vi "Guitar SubviUpdated.vi"(0 "error out":errorcluster, 1 "Image Dst Out":T2) -> (11 "Orange Guitar LED":bool, 13 "Red Guitar LED":bool, 15 "Green Guitar LED":bool, 23 "Blue Guitar LED":bool, 24 "Yellow Guitar LED":bool)   [LabVIEW 2009]
uses:
  <vilib>/vision/Image Controls.llb/IMAQ Image.ctl
  <vilib>/Analysis/3filter.llb/Filter Passband Type.ctl
  <vilib>/Analysis/3filter.llb/Butterworth Filter (DBL).vi
  <vilib>/Analysis/NI_AALBase.lvlib
  <vilib>/vision/NI_Vision_Development_Module.lvlib
panel:
  in  "Yellow Guitar":T1={"Global Rectangle"=[40, 272, 657, 396], "Contours"=[{"ID"=enum."External", "Type"=3, "Coordinates"=[40, 272, 657, 396]}]} {"Contours"."Type" items=["No Selection", "Point", "Line", "Rectangle", "Oval", "Polygon", "Freehand Region", "Annulus", "Unused2", "Unused3", "Broken Line", "Freehand Line", "Rotated Rectangle"]}
  in  "Red Guitar":T1={"Global Rectangle"=[40, 272, 657, 396], "Contours"=[{"ID"=enum."External", "Type"=3, "Coordinates"=[40, 272, 657, 396]}]} {"Contours"."Type" items=["No Selection", "Point", "Line", "Rectangle", "Oval", "Polygon", "Freehand Region", "Annulus", "Unused2", "Unused3", "Broken Line", "Freehand Line", "Rotated Rectangle"]}
  in  "Orange Guitar":T1={"Global Rectangle"=[40, 272, 657, 396], "Contours"=[{"ID"=enum."External", "Type"=3, "Coordinates"=[40, 272, 657, 396]}]} {"Contours"."Type" items=["No Selection", "Point", "Line", "Rectangle", "Oval", "Polygon", "Freehand Region", "Annulus", "Unused2", "Unused3", "Broken Line", "Freehand Line", "Rotated Rectangle"]}
  in  "Green Guitar":T1={"Global Rectangle"=[40, 272, 657, 396], "Contours"=[{"ID"=enum."External", "Type"=3, "Coordinates"=[40, 272, 657, 396]}]} {"Contours"."Type" items=["No Selection", "Point", "Line", "Rectangle", "Oval", "Polygon", "Freehand Region", "Annulus", "Unused2", "Unused3", "Broken Line", "Freehand Line", "Rotated Rectangle"]}
  in  "Blue Guitar":T1={"Global Rectangle"=[40, 272, 657, 396], "Contours"=[{"ID"=enum."External", "Type"=3, "Coordinates"=[40, 272, 657, 396]}]} {"Contours"."Type" items=["No Selection", "Point", "Line", "Rectangle", "Oval", "Polygon", "Freehand Region", "Annulus", "Unused2", "Unused3", "Broken Line", "Freehand Line", "Rotated Rectangle"]}
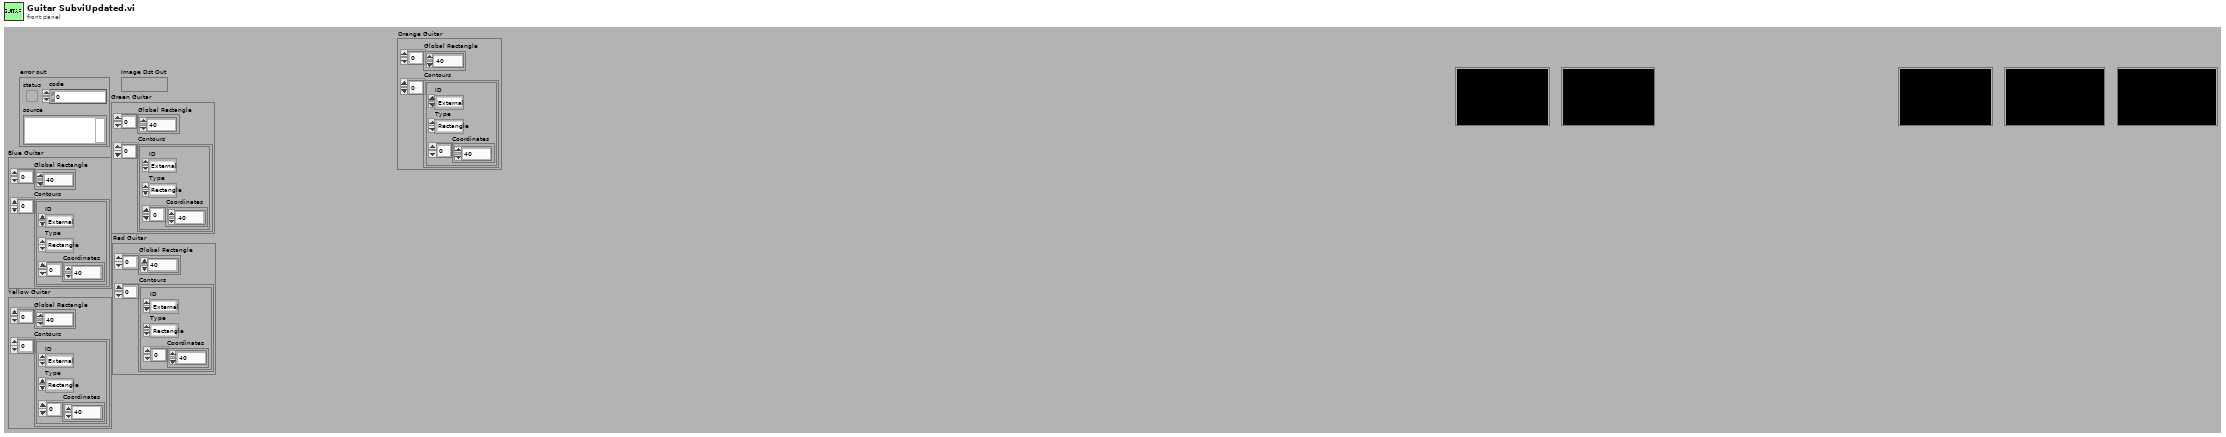
[diagram p1: front panel]
types:
  T1 = cluster{"Global Rectangle":i32[], "Contours":cluster{"ID":enum32{"External", "Internal"}, "Type":u32, "Coordinates":i32[]}[]}
  T2 = typedef "IMAQ Image.ctl" = refnum<image>
  T3 = typedef "NI_AALBase.lvlib/Filter Passband Type.ctl" = enum32{"Lowpass", "Highpass", "Bandpass", "Bandstop"}
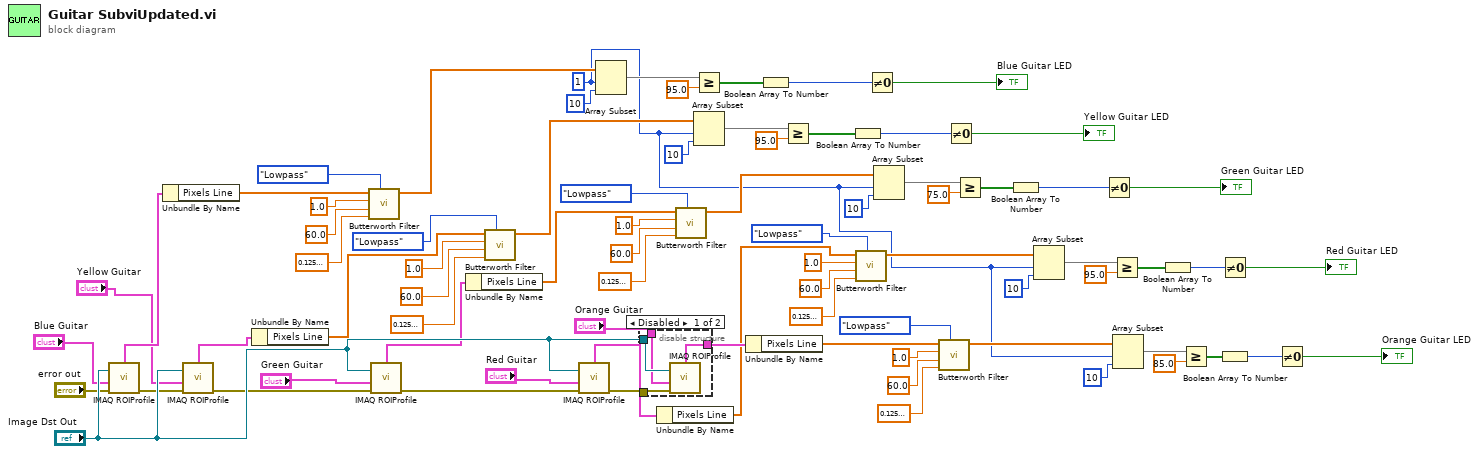
[diagram p0: block diagram]
diagram:
  w6 = 1 ("index")
  n1 = call "IMAQ ROIProfile"("error in (no error)"="error out", "ROI Descriptor"="Blue Guitar", "Image"="Image Dst Out") -> ("error out"=w47:errorcluster, "ROI Graph"=w46:cluster{"x0":sgl, "dx":sgl, "Pixels Line":sgl[]})  [unwired: 4 out]
  n2 = Unbundle By Name(w46) -> ("Pixels Line"=w67:sgl[])
  n3 = call "IMAQ ROIProfile"("error in (no error)"=w47, "ROI Descriptor"="Yellow Guitar", "Image"="Image Dst Out") -> ("error out"=w19:errorcluster, "ROI Graph"=w50:cluster{"x0":sgl, "dx":sgl, "Pixels Line":sgl[]})  [unwired: 4 out]
  n4 = Unbundle By Name(w50) -> ("Pixels Line"=w53:sgl[])
  n5 = call-poly <vilib>:"Butterworth Filter.vi"("filter type"=Filter_Passband_Type."Lowpass", "low cutoff freq: fl"=0.12500000000000006 ("low 3"), "high cutoff freq: fh"=60.0 ("high 14"), "sampling freq: fs"=1.0 ("sampling  9"), "X"=w67) -> ("Filtered X"=w33:dbl[])  [unwired: 3 in, 1 out]
  n6 = call "IMAQ ROIProfile"("error in (no error)"=w19, "ROI Descriptor"="Green Guitar", "Image"="Image Dst Out") -> ("error out"=w20:errorcluster, "ROI Graph"=w44:cluster{"x0":sgl, "dx":sgl, "Pixels Line":sgl[]})  [unwired: 4 out]
  n7 = Unbundle By Name(w44) -> ("Pixels Line"=w41:sgl[])
  n8 = call-poly <vilib>:"Butterworth Filter.vi"("filter type"=Filter_Passband_Type."Lowpass", "low cutoff freq: fl"=0.12500000000000006 ("low  12"), "high cutoff freq: fh"=60.0 ("high 13"), "sampling freq: fs"=1.0 ("sampling 12"), "X"=w53) -> ("Filtered X"=w49:dbl[])  [unwired: 3 in, 1 out]
  n9 = call "IMAQ ROIProfile"("error in (no error)"=w20, "ROI Descriptor"="Red Guitar", "Image"="Image Dst Out") -> ("error out"=w71:errorcluster, "ROI Graph"=w22:cluster{"x0":sgl, "dx":sgl, "Pixels Line":sgl[]})  [unwired: 4 out]
  n10 = Array Subset(array=w33, index=w6, length=10) -> (w62:dbl[])
  n11 = disable-structure shown="Disabled" {
    disable-tunnel: [w81 _] -> w72
    disable-tunnel: w71 -> [w80 _]
    disable-tunnel: "Image Dst Out" -> [w79 _]
    disable-tunnel: "Orange Guitar" -> [w78 _]
    frame #0 {
      n12 = call "IMAQ ROIProfile"("error in (no error)"=w80, "ROI Descriptor"=w78, "Image"=w79) -> ("ROI Graph"=w81:cluster{"x0":sgl, "dx":sgl, "Pixels Line":sgl[]})  [unwired: 5 out]
    }
    frame #1 {
    }
  }
  n13 = Unbundle By Name(w22) -> ("Pixels Line"=w25:sgl[])
  n14 = call-poly <vilib>:"Butterworth Filter.vi"("filter type"=Filter_Passband_Type."Lowpass", "low cutoff freq: fl"=0.12500000000000006 ("low  11"), "high cutoff freq: fh"=60.0 ("high 12"), "sampling freq: fs"=1.0 ("sampling 11"), "X"=w41) -> ("Filtered X"=w45:dbl[])  [unwired: 3 in, 1 out]
  n15 = Greater Or Equal?(x=w62, y=95.0) -> (x >= y?=w7:bool[])
  n16 = Array Subset(array=w49, index=w6, length=10) -> (w58:dbl[])
  n17 = Unbundle By Name(w72) -> ("Pixels Line"=w15:sgl[])
  n18 = Boolean Array To Number(Boolean array=w7) -> (number=w60:u32)
  n19 = Greater Or Equal?(x=w58, y=95.0) -> (x >= y?=w56:bool[])
  n20 = Boolean Array To Number(Boolean array=w56) -> (number=w55:u32)
  n21 = call-poly <vilib>:"Butterworth Filter.vi"("filter type"=Filter_Passband_Type."Lowpass", "low cutoff freq: fl"=0.12500000000000006 ("low  10"), "high cutoff freq: fh"=60.0 ("high 11"), "sampling freq: fs"=1.0 ("sampling 10"), "X"=w25) -> ("Filtered X"=w21:dbl[])  [unwired: 3 in, 1 out]
  n22 = Not Equal To 0?(x=w60) -> (x != 0?=→"Blue Guitar LED":bool)
  n23 = Array Subset(array=w45, index=w6, length=10) -> (w36:dbl[])
  n24 = call-poly <vilib>:"Butterworth Filter.vi"("filter type"=Filter_Passband_Type."Lowpass", "low cutoff freq: fl"=0.12500000000000006 ("low  9"), "high cutoff freq: fh"=60.0 ("high 10"), "sampling freq: fs"=1.0 ("sampling 9"), "X"=w15) -> ("Filtered X"=w18:dbl[])  [unwired: 3 in, 1 out]
  n25 = Not Equal To 0?(x=w55) -> (x != 0?=→"Yellow Guitar LED":bool)
  n26 = Greater Or Equal?(x=w36, y=75.0) -> (x >= y?=w38:bool[])
  n27 = Boolean Array To Number(Boolean array=w38) -> (number=w39:u32)
  n28 = Array Subset(array=w21, index=w6, length=10) -> (w30:dbl[])
  n29 = Not Equal To 0?(x=w39) -> (x != 0?=→"Green Guitar LED":bool)
  n30 = Greater Or Equal?(x=w30, y=95.0) -> (x >= y?=w28:bool[])
  n31 = Array Subset(array=w18, index=w6, length=10) -> (w10:dbl[])
  n32 = Boolean Array To Number(Boolean array=w28) -> (number=w27:u32)
  n33 = Greater Or Equal?(x=w10, y=85.0) -> (x >= y?=w12:bool[])
  n34 = Not Equal To 0?(x=w27) -> (x != 0?=→"Red Guitar LED":bool)
  n35 = Boolean Array To Number(Boolean array=w12) -> (number=w13:u32)
  n36 = Not Equal To 0?(x=w13) -> (x != 0?=→"Orange Guitar LED":bool)
